vi "Convert Field Value.vi"(8 "error in":errorcluster, 11 "Field Value":variant) -> (0 "error out":errorcluster, 3 "Field String":string)   [LabVIEW 2020, in "InfluxDB v2 Client.lvlib"]
doc: "Converts a filed value (variant) depending on data type into string for using in the line protocol"
uses:
  InfluxDB v2 Client.lvlib
  <vilib>/Utility/Data Type/NI_Data Type.lvlib
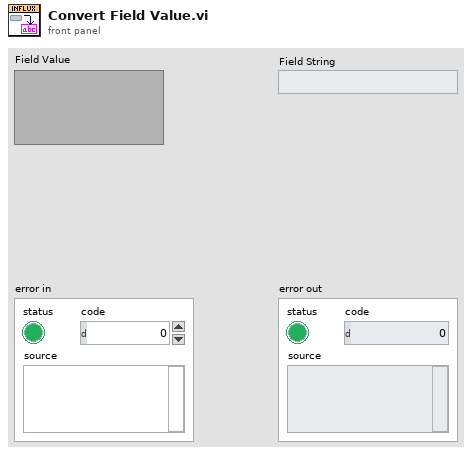
[diagram p1: front panel]
types:
  T1 = typedef "NI_Data Type.lvlib/Data Type.ctl" = enum8{"Invalid Type", "Void", "I8", "I16", "I32", "I64", "U8", "U16", "U32", "U64", "Single Float", "Double Float", "Extended Float", "Single Complex", "Double Complex", "Extended Complex", "Enum U8", "Enum U16", "Enum U32", "Enum U64", "Single Float With Unit", "Double Float With Unit", "Extended Float With Unit", "Single Complex with Unit", "Double Complex with Unit", "Extended Complex with Unit", "Boolean", "String", "Path", "Picture", "Tag", "Array", "Cluster", "Variant", "LV Variant", "Waveform", "Timestamp", "Digital Waveform", "Digital Data", "ExpressData", "Refnum", "External Data", "VI", "Poly VI", "LabVIEW Class Instance", "Fixed Point", "Set Collection", "Map Collection"}
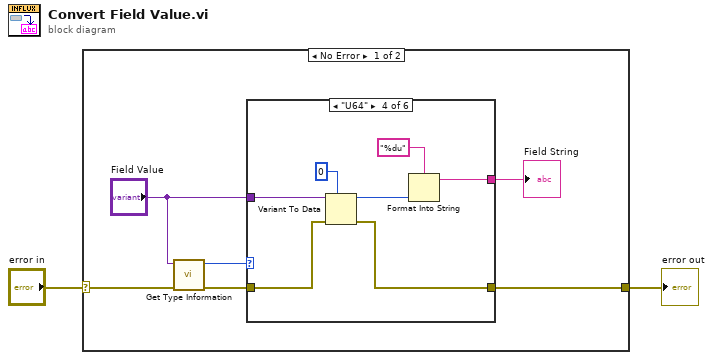
[diagram p0: block diagram]
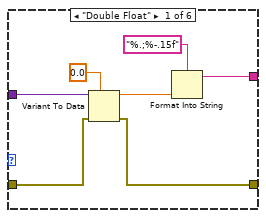
[diagram p2: hidden frame]
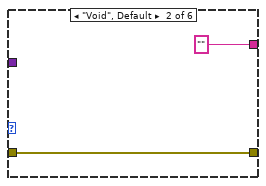
[diagram p3: hidden frame]
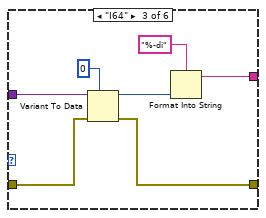
[diagram p4: hidden frame]
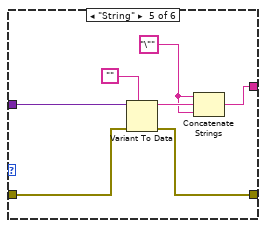
[diagram p5: hidden frame]
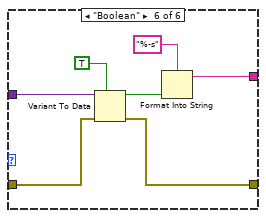
[diagram p6: hidden frame]
diagram:
  n1 = case shown="No Error" "error in" {
    selector: "error in" -> [w5 w46]
    tunnel: [w3 w46] -> w1
    frame No Error {
      n2 = call <vilib>:"Get Type Information.vi"("error in (no error)"=w5, "variant"="Field Value") -> ("error out"=w4:errorcluster, "type"=w8:T1)  [unwired: 5 in, 3 out]
      n3 = case shown="\"U64\"" w8 {
        tunnel: [w12 "" w21 w28 w32 w42] -> w7
        tunnel: "Field Value" -> [w11 _ w20 w27 w37 w41]
        tunnel: w4 -> [w10 w17 w19 w26 w36 w40]
        tunnel: [w9 w17 w18 w25 w35 w39] -> w3
        frame "Double Float" {
          n4 = Variant To Data(error in=w10, type=0.0, Variant=w11) -> (data=w14:dbl, error out=w9:errorcluster)
          n5 = Format Into String(format string="%.;%-.15f", w14) -> (resulting string=w12:string)  [unwired: 2 in, 1 out]
        }
        frame "Void", Default {
        }
        frame "I64" {
          n6 = Variant To Data(error in=w19, type=i64 0, Variant=w20) -> (data=w22:i64, error out=w18:errorcluster)
          n7 = Format Into String(format string="%-di", w22) -> (resulting string=w21:string)  [unwired: 2 in, 1 out]
        }
        frame "U64" {
          n8 = Variant To Data(error in=w26, type=u64 0, Variant=w27) -> (data=w29:u64, error out=w25:errorcluster)
          n9 = Format Into String(format string="%du", w29) -> (resulting string=w28:string)  [unwired: 2 in, 1 out]
        }
        frame "String" {
          w33 = "\""
          n10 = Variant To Data(error in=w36, type="", Variant=w37) -> (data=w34:string, error out=w35:errorcluster)
          n11 = Concatenate Strings(w33, w34, w33) -> (w32:string)
        }
        frame "Boolean" {
          n12 = Variant To Data(error in=w40, type=TRUE, Variant=w41) -> (data=w44:bool, error out=w39:errorcluster)
          n13 = Format Into String(format string="%-s", w44) -> (resulting string=w42:string)  [unwired: 2 in, 1 out]
        }
      }
      "Field String" <- w7
    }
    frame Error {
    }
  }
  "error out" <- w1
